vi "getScriptName.vi"(8 "error in (no error)":errorcluster, 11 "FileNeologist.lvclass in":refnum<class "FileNeologist.lvclass">) -> (0 "error out":errorcluster, 2 "scriptName":string, 3 "FileNeologist.lvclass out":refnum<class "FileNeologist.lvclass">)   [LabVIEW 2009, in "Tools.lvlib" / "Filing.lvlib" / "FileNeologist.lvclass"]
uses:
  FileNeologist.lvclass
  FileNeologist.lvclass/FileNeologist.ctl
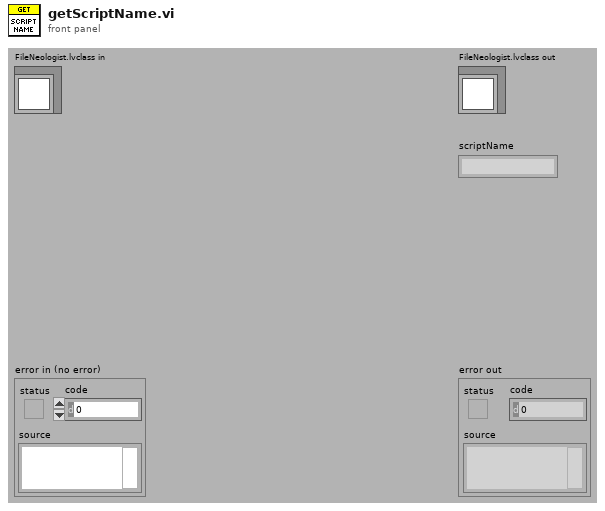
[diagram p1: front panel]
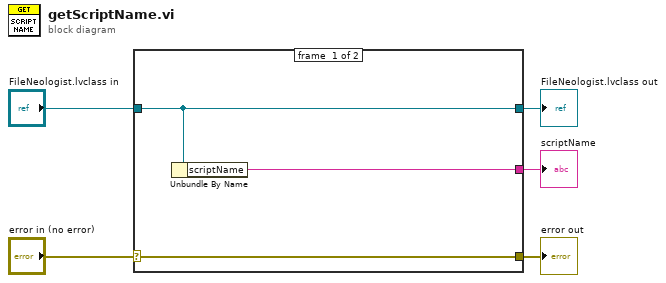
[diagram p0: block diagram]
diagram:
  n1 = case shown="No Error" "error in (no error)" {
    selector: "error in (no error)" -> [w8 w9]
    tunnel: [w8 w9] -> w4
    tunnel: [w7 w10] -> w2
    tunnel: "FileNeologist.lvclass in" -> [w7 w10]
    tunnel: [w6 _] -> w1
    frame #0 {
      n2 = Unbundle By Name(w7) -> ("scriptName"=w6:string)
    }
    frame #1 {
    }
  }
  "error out" <- w4
  "FileNeologist.lvclass out" <- w2
  "scriptName" <- w1
